vi "Acquire.vi"(8 "error in (no error)":errorcluster, 9 "?":T3 {"Image Type" items=["Grayscale (U8)", "Grayscale (I16)", "Grayscale (SGL)", "Complex (CSG)", "RGB (U32)", "HSL (U32)", "RGB (U64)", "Grayscale (U16)"]}, 10 "Settings":T5={"Harware Configuration"={"Camera"="cam1", "Frames Per Second"=15, "Simulate Recording"=FALSE, "Simulated Recording Sample"=path "", "Timestamp Method"=enum."Camera Timestamp"}, "Base Recording Path"=path "", "Type Of Recording"="", "Recording Codec"="", "TrackingSettings"={"Max Radius"=0, "Threshold"=160.0, "ROI"={"Left"=0, "Top"=0, "Right"=0, "Bottom"=0, "Rotation"=0.0}}, "Calibration"={"Pixel Width (X)"=1.0, "Pixel Height (Y)"=1.0}, "Broadcast Length"=0} {"Broadcast Length" min=0; "TrackingSettings"."ROI"."Rotation" format="%.2f"; "TrackingSettings"."ROI"."Left" scale=0.0..1024.0; "TrackingSettings"."ROI"."Right" scale=0.0..1024.0; "TrackingSettings"."Threshold" scale=0.0..255.0}, 11 "Acquired Data":T1 {"Frame Data"."Image Type" items=["Grayscale (U8)", "Grayscale (I16)", "Grayscale (SGL)", "Complex (CSG)", "RGB (U32)", "HSL (U32)", "RGB (U64)", "Grayscale (U16)"]}) -> (0 "error out":errorcluster, 1 "Acquisition Object":T3 {"Image Type" items=["Grayscale (U8)", "Grayscale (I16)", "Grayscale (SGL)", "Complex (CSG)", "RGB (U32)", "HSL (U32)", "RGB (U64)", "Grayscale (U16)"]}, 3 "Acquired Data out":T1 {"Frame Data"."Image Type" items=["Grayscale (U8)", "Grayscale (I16)", "Grayscale (SGL)", "Complex (CSG)", "RGB (U32)", "HSL (U32)", "RGB (U64)", "Grayscale (U16)"]})   [LabVIEW 2017, in "ImageAcquisitionLibrary.lvlib"]
uses:
  ImageAcquisitionLibrary.lvlib
  Settings/Settings.ctl
  <vilib>/userdefined/High Color/IMAQdx.ctl
  Tracking/TrackingSettings.ctl
  Settings/Calibration.ctl
  AcquisitionObject.ctl
  <vilib>/vision/Image Controls.llb/IMAQ Image.ctl
  AcquireData.ctl
  <vilib>/vision/driver/NI_Vision_Acquisition_Software.lvlib
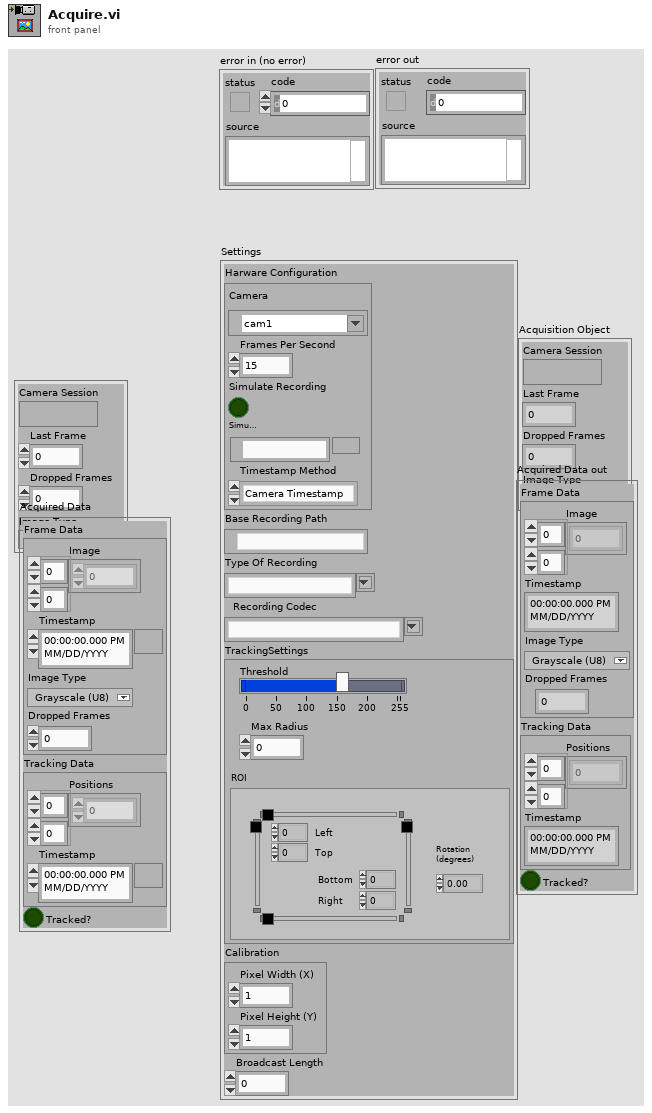
[diagram p1: front panel]
types:
  T1 = typedef "ImageAcquisitionLibrary.lvlib/AcquireData.ctl" = cluster{"Frame Data":cluster{"Image":u32[][], "Timestamp":timestamp, "Image Type":T2, "Dropped Frames":u32}, "Tracking Data":cluster{"Positions":dbl[][], "Timestamp":timestamp}, "Tracked?":bool}
  T2 = typedef "Image Type" = u32
  T3 = typedef "ImageAcquisitionLibrary.lvlib/AcquisitionObject.ctl" = cluster{"Camera Session":T4, "Last Frame":u32, "Dropped Frames":u32, "Image Type":T2}
  T4 = typedef "IMAQ Image.ctl" = refnum<image>
  T5 = typedef "ImageAcquisitionLibrary.lvlib/Settings.ctl" = cluster{"Harware Configuration":cluster{"Camera":T6, "Frames Per Second":u32, "Simulate Recording":bool, "Simulated Recording Sample":path, "Timestamp Method":enum16{"System Timestamp", "Camera Timestamp", "IMAQdx Timestamp"}}, "Base Recording Path":path, "Type Of Recording":string, "Recording Codec":string, "TrackingSettings":T7, "Calibration":T9, "Broadcast Length":i32}
  T6 = typedef "IMAQdx.ctl" = refnum<k21>
  T7 = typedef "ImageAcquisitionLibrary.lvlib/TrackingSettings.ctl" = cluster{"Max Radius":i32, "Threshold":sgl, "ROI":T8}
  T8 = typedef "IMAQ Rectangle" = cluster{"Left":i32, "Top":i32, "Right":i32, "Bottom":i32, "Rotation":dbl}
  T9 = typedef "ImageAcquisitionLibrary.lvlib/Calibration.ctl" = cluster{"Pixel Width (X)":dbl, "Pixel Height (Y)":dbl}
  T10 = enum16{"System Timestamp", "Camera Timestamp", "IMAQdx Timestamp"}
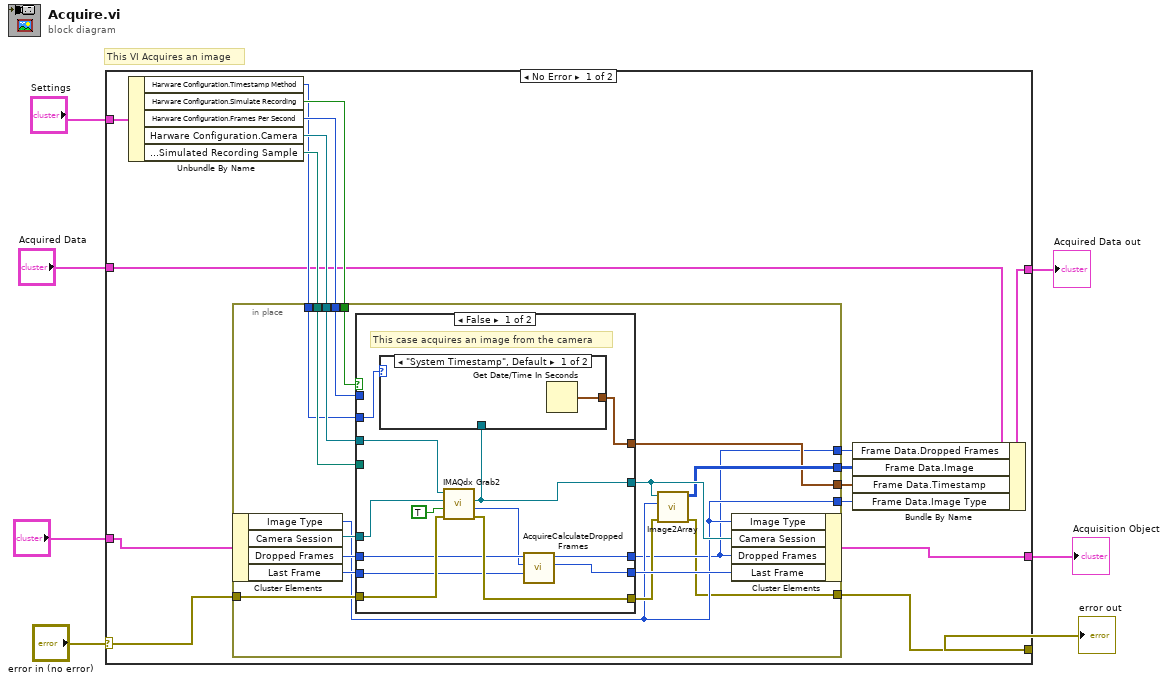
[diagram p0: block diagram]
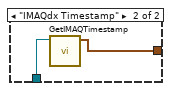
[diagram p2: hidden frame]
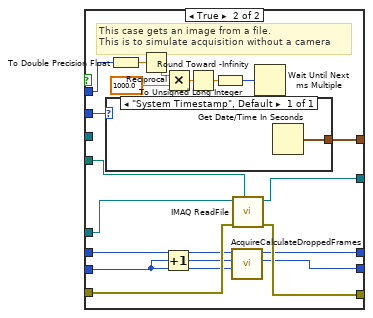
[diagram p3: hidden frame]
diagram:
  # "This VI Acquires an image"
  n1 = case shown="No Error" "error in (no error)" {
    selector: "error in (no error)" -> [w18 w79]
    tunnel: "Acquired Data" -> [w14 w78]
    tunnel: "Settings" -> [w23 _]
    tunnel: [w17 w79] -> w6
    tunnel: [w12 w78] -> w1
    tunnel: "?" -> [w15 w77]
    tunnel: [w11 w77] -> w3
    frame No Error {
      n2 = Unbundle By Name(w23) -> ("Harware Configuration.Timestamp Method"=w16:T10, "Harware Configuration.Simulate Recording"=w22:bool, "Harware Configuration.Frames Per Second"=w21:u32, "Harware Configuration.Camera"=w20:T6, "Harware Configuration.Simulated Recording Sample"=w19:path)
      n3 = in-place {
        in-place-border: w18 -> [w40]
        in-place-border: w22 -> [w39]
        in-place-border: [w24] -> w17
        in-place-border: w21 -> [w38]
        in-place-border: w20 -> [w36]
        in-place-border: w19 -> [w37]
        in-place-border: w16 -> [w35]
        in-place-border: [w28] -> w13
        in-place-border: [w27] -> w10
        in-place-border: [w26] -> w9
        in-place-border: [w25] -> w8
        n4 = in-place-cluster #1(w15) -> ("Image Type"=w27:T2, "Camera Session"=w34:T4, "Dropped Frames"=w33:u32, "Last Frame"=w31:u32)
        n5 = case shown="False" w39 {
          tunnel: w40 -> [w52 w75]
          tunnel: [w51 w74] -> w30
          tunnel: w33 -> [w50 w63]
          tunnel: w31 -> [w49 w66]
          tunnel: [w45 w64] -> w29
          tunnel: [w48 w65] -> w32
          tunnel: w37 -> [_ w61]
          tunnel: w38 -> [_ w62]
          tunnel: w36 -> [w44 _]
          tunnel: w35 -> [w47 w60]
          tunnel: [w46 w59] -> w26
          tunnel: w34 -> [w43 w58]
          tunnel: [w41 w57] -> w25
          frame False {
            # "This case acquires an image from the camera"
            n6 = call <vilib>:"IMAQdx Grab2.vi"("error in"=w52, "Wait for Next Buffer? (Yes)"=TRUE, "Image In"=w43, "Session In"=w44) -> ("error out"=w51:errorcluster, "Buffer Number Out"=w42:u32, "Image Out"=w45:T4)  [unwired: 4 in, 1 out]
            n7 = case shown="\"System Timestamp\", Default" w47 {
              tunnel: [w54 w56] -> w46
              tunnel: w45 -> [_ w55]
              frame "System Timestamp", Default {
                n8 = Get Date/Time In Seconds() -> (seconds since 1Jan1904=w54:timestamp)
              }
              frame "IMAQdx Timestamp" {
                n9 = call "GetIMAQTimestamp.vi"("Refnum in"=w55) -> ("Time Stamp"=w56:timestamp)  [unwired: 10 in]
              }
            }
            n10 = call "AcquireCalculateDroppedFrames.vi"("LastBuffer"=w49, "CurrentBuffer"=w42, "DroppedFrames"=w50) -> ("CurrentBufferOut"=w48:u32, "DroppedOut"=w41:u32)  [unwired: 7 in]
          }
          frame True {
            # "This case gets an image from a file. \nThis is to simulate acquisition without a camera"
            n11 = case shown="\"System Timestamp\", Default" w60 {
              tunnel: [w76] -> w59
              frame "System Timestamp", Default {
                n12 = Get Date/Time In Seconds() -> (seconds since 1Jan1904=w76:timestamp)
              }
            }
            n13 = To Double Precision Float(number=w62) -> (double precision float=w73:dbl)
            n14 = Reciprocal(x=w73) -> (1/x=w72:dbl)
            n15 = Increment(x=w66) -> (x+1=w67:u32)
            n16 = Multiply(x=w72, y=1000.0) -> (x*y=w70:dbl)
            n17 = Round Toward -Infinity(1:w70) -> (0:w68:dbl)
            n18 = To Unsigned Long Integer(number=w68) -> (unsigned 32bit integer=w69:u32)
            n19 = call "AcquireCalculateDroppedFrames.vi"("LastBuffer"=w66, "CurrentBuffer"=w67, "DroppedFrames"=w63) -> ("CurrentBufferOut"=w65:u32, "DroppedOut"=w57:u32)  [unwired: 7 in]
            n20 = call "IMAQ ReadFile"("File Path"=w61, "error in (no error)"=w75, "Image"=w58) -> ("error out"=w74:errorcluster, "Image Out"=w64:T4)  [unwired: 4 in, 3 out]
            n21 = Wait Until Next ms Multiple(millisecond multiple=w69) -> ()  [unwired: 1 out]
          }
        }
        n22 = call "Image2Array.vi"("error in (no error)"=w30, "Image Type"=w27, "Image"=w29) -> ("error out"=w24:errorcluster, "Image Pixels (U32)"=w28:u32[][])  [unwired: 7 in]
        n23 = in-place-cluster #1("Image Type"=w27, "Camera Session"=w29, "Dropped Frames"=w25, "Last Frame"=w32) -> (w11:T3)
      }
      n24 = Bundle By Name(cluster=w14, "Frame Data.Dropped Frames"=w8, "Frame Data.Image"=w13, "Frame Data.Timestamp"=w9, "Frame Data.Image Type"=w10) -> (w12:T1)
    }
    frame Error {
    }
  }
  "error out" <- w6
  "Acquisition Object" <- w3
  "Acquired Data out" <- w1
